vi "Dashboard Main.vi"() -> ()   [LabVIEW 2013]
uses:
  <vilib>/event_ctls.llb/eventvkey.ctl
  <vilib>/Rock Robotics/WPI/Dashboard/WPI_DashboardLogging Global.vi
  <vilib>/Utility/config.llb/Write Key (String).vi
  <vilib>/Utility/config.llb/Write Key (I32).vi
  <vilib>/Utility/config.llb/NI_LVConfig.lvlib
panel:
  out "fps":dbl format="%#.1g"
  out "Mbps":dbl format="%#.1g"
  out "Mbps 2":bool
  in  "DB Camera Config":bool
  out "Image Message":string="Timeout in Camera Communications"
  in  "Rec Mode":enum32{"Stop", "Record", "Playback"}(radio)
  in  "Dashboard Tab":T1(tab)
  in  "Encoder":dbl
  out "Compressor On/Off":bool
  in  "Camera Settings":T2={"Frame Rate"=30, "Compression"=30, "Size"=1} {"Frame Rate" scale=1.0..30.0; "Size" items=["640x480", "320x240", "160x120"]}
  out "MotorSliders R":cluster{"MotorSlide1":dbl, "MotorSlide2":dbl} {"MotorSlide2" scale=-1.0..1.0 scale format="%#_2e"; "MotorSlide1" scale=-1.0..1.0 scale format="%#_2e"}
  out "MotorChart R":cluster{"Numeric":dbl, "Numeric":dbl}(graph)
  out "MotorSliders L":T3 {"MotorSlide4 2" scale=0.0..14.0 scale format="%#_2e"; "MotorSlide2" scale=-1.0..1.0 scale format="%#_2e"; "MotorSlide1" scale=-1.0..1.0 scale format="%#_2e"}
  out "MotorChart L":T4(graph)
  out "JS1 Z":dbl(slide) scale=-1.0..1.0 scale format="%#_2e"
  out "Joystick 1":cluster{"X":dbl, "Y":dbl}[](graph)
  out "JS Buttons 1":T5
  out "JS2 Z":dbl(slide) scale=-1.0..1.0 scale format="%#_2e"
  out "Joystick 2":cluster{"X":dbl, "Y":dbl}[](graph)
  out "JS Buttons 2":T5
  out "Mode":T6(ring)=enum."Auto Disabled"
  out "Camera IP":string
  out "LED 1":bool
  in  "Throttle":dbl
  in  "Slider 1":dbl(slide) scale=0.0..100.0
  in  "Checkbox 2":bool
  in  "Checkbox 1":bool
  in  "Test Slider":dbl(slide) scale=0.0..100.0 scale format="%#_3g"
  in  "On/Off":bool caption="Solenoid"
  in  "Test Name":u16(ring) items=["Select the test to run...", "Example Test", "-------------------------------", "List of tests is built in robot code.", "Replace with your own automated tests."]
  in  "Test Tree":string(tree)
  in  "Motor":cluster{"Value":dbl, "Enable":bool} {"Value" scale=-1.0..1.0 scale format="%#_3g"}
  out "Progress":T7 {"Test Progress" scale=0.0..100.0}
  in  "Rev/Fwd":cluster{"Forward":bool, "Reverse":bool}
  in  "Test Ring":u16(ring) items=["Auto", "Fixed indoor", "Fixed outdoor 1", "Fixed outdoor 2", "Fixed fluorescent 1", "Fixed fluorescent 2", "Hold current"]
  in  "Listbox":i32(listbox)
  out "Tree":string(tree)
  out "Camera Image":T8(plugin-control)
  in  "Enable":bool
  # "Left"
  # "Front"
  # "Right"
  # "Battery"
  # "Customize by placing controls and indicators here and name to\nmatch Dashboard Variables on robot."
  # "This tab is a great place for autonomous settings and validation.\nCustomize by placing controls and indicators here and name to\nmatch Dashboard Variables on robot."
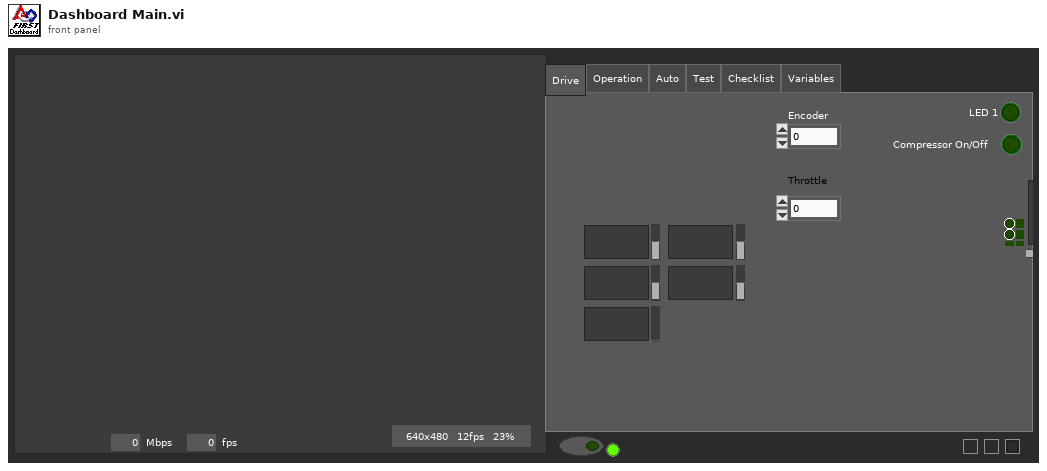
[diagram p1: front panel]
types:
  T1 = enum32{"Drive", "Operation", "Auto", "Test", "Checklist", "Variables"}
  T2 = cluster{"Frame Rate":i32, "Compression":i32, "Size":u16}
  T3 = cluster{"MotorSlide1":dbl, "MotorSlide2":dbl, "MotorSlide4 2":dbl}
  T4 = cluster{"Numeric":dbl, "Numeric":dbl, "Battery":sgl}
  T5 = cluster{bool, bool, bool, bool, bool, bool, bool, bool, bool, bool, bool, bool}
  T6 = enum8{"Tele-Op Disabled", "Tele-Op Enabled", "Auto Disabled", "Auto Enabled", "Test Disabled", "Test Enabled", ""}
  T7 = cluster{"Test Progress":u8, "Test Progress Text":string}
  T8 = typedef "IMAQ Image.ctl" = refnum<image>
  T9 = typedef "Image Type" = u32
  T10 = cluster{"Digital Inputs":bool[], "Digital Outputs":bool[]}
  T11 = cluster{"Competition mode":bool, "Robot Link":bool, "Autonomous":bool, "Enabled":bool, "E-Stop":bool, "Simulated":bool, "TestMode":bool, "Docked Window":bool}
  T12 = cluster{"Boolean Array[0]":bool, "Boolean Array[1]":bool, "Boolean Array[2]":bool, "Boolean Array[3]":bool, "Boolean Array[4]":bool, "Boolean Array[5]":bool, "Boolean Array[6]":bool, "Boolean Array[7]":bool, "Boolean Array[8]":bool, "Boolean Array[9]":bool, "Boolean Array[10]":bool, "Boolean Array[11]":bool}
  T13 = typedef "NI_LVConfig.lvlib/Config Data RefNum.ctl" = refnum<k1>
  T14 = typedef "eventvkey.ctl" = enum16{"ASCII", "Enter", "Return", "Shift", "Ctrl", "Alt", "Cmd", "Opt", "Caps", "NumLock", "Clear", "Break", "Up", "Down", "Left", "Right", "Insert", "Delete", "Home", "End", "PageUp", "PageDown", "Escape", "Help", "Pause", "ScrollLock", "F1", "F2", "F3", "F4", "F5", "F6", "F7", "F8", "F9", "F10", "F11", "F12", "F13", "F14", "F15", "F16", "F17", "F18", "F19", "F20", "F21", "F22", "F23", "F24", "Play", "VolumeUp", "VolumeDown", "Mute", "Two Byte Char"}
  T15 = cluster{"Image Size":bool, "Image Type":bool, "Pixel Value":bool, "ROI Information":bool, "Zoom Factor":bool}
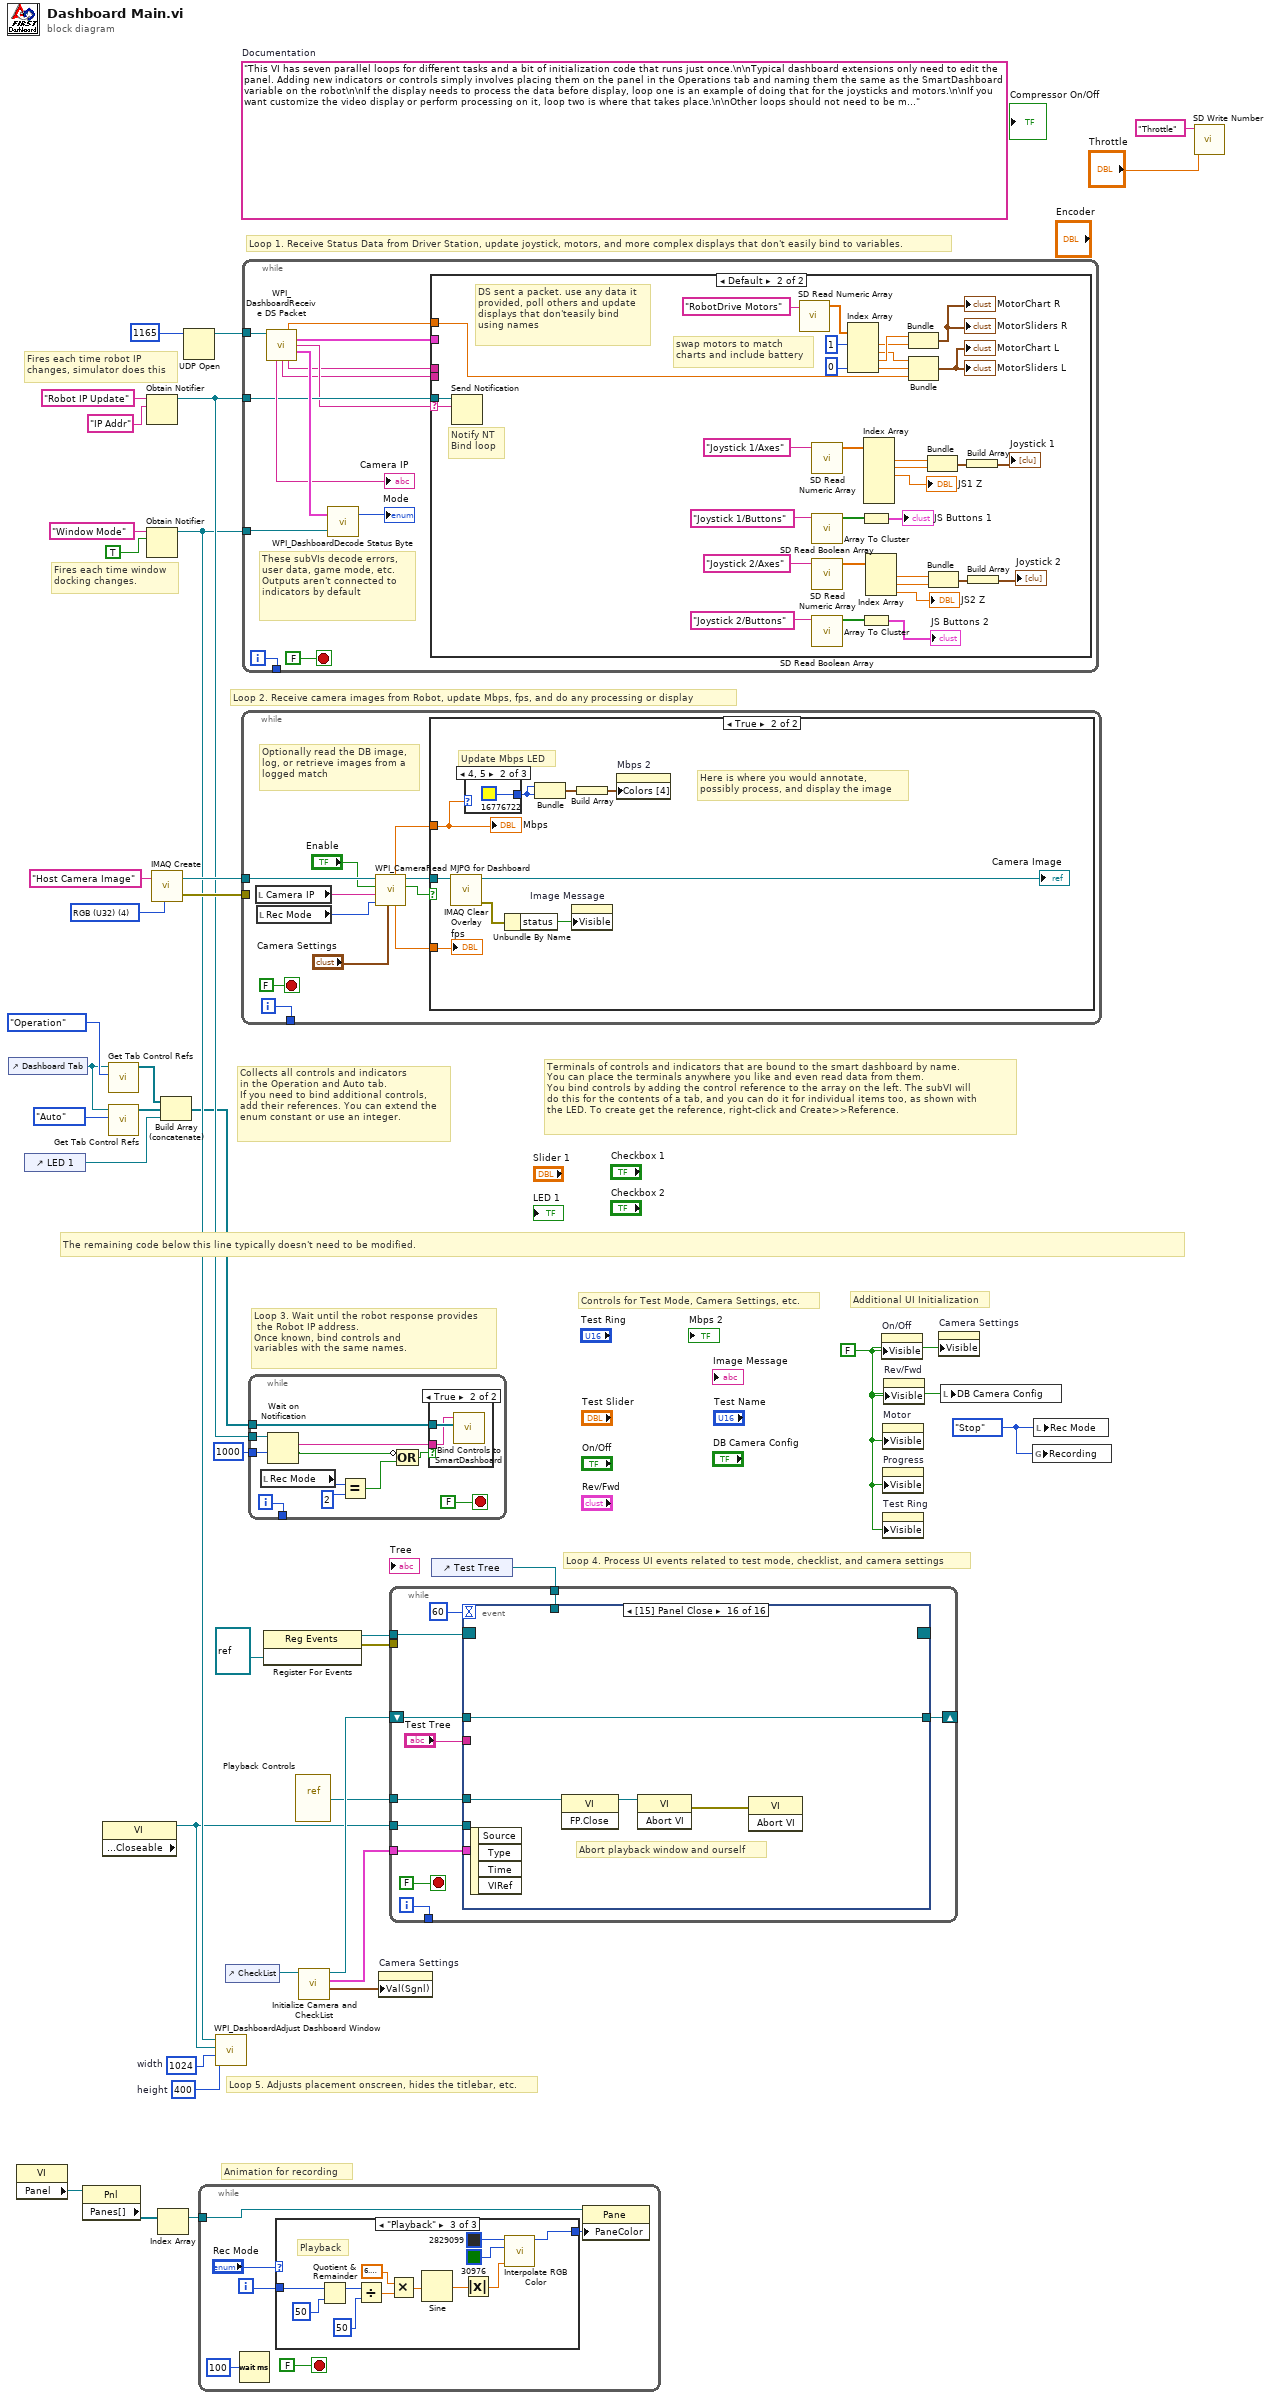
[diagram p0: block diagram]
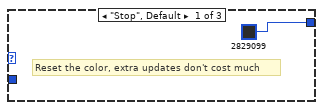
[diagram p2: hidden frame]
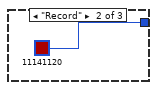
[diagram p3: hidden frame]
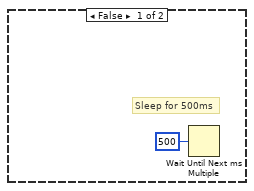
[diagram p5: hidden frame]
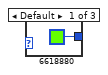
[diagram p6: hidden frame]
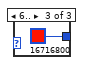
[diagram p7: hidden frame]
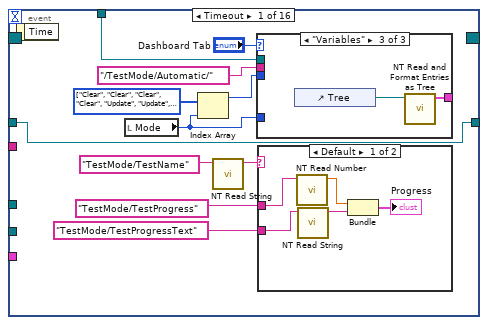
[diagram p8: hidden frame]
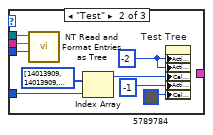
[diagram p10: hidden frame]
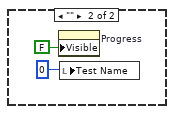
[diagram p11: hidden frame]
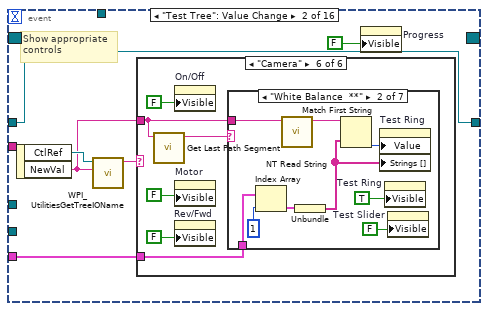
[diagram p12: hidden frame]
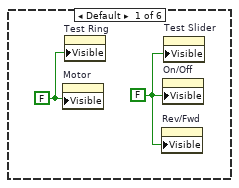
[diagram p13: hidden frame]
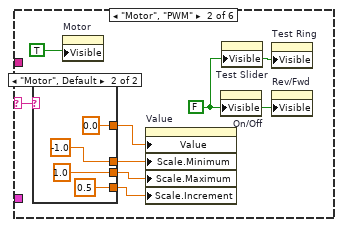
[diagram p14: hidden frame]
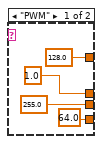
[diagram p15: hidden frame]
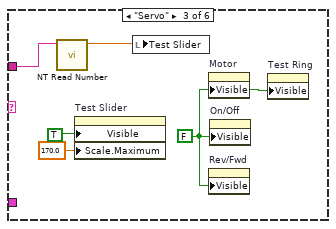
[diagram p16: hidden frame]
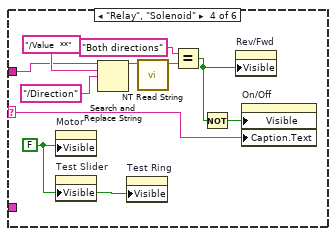
[diagram p17: hidden frame]
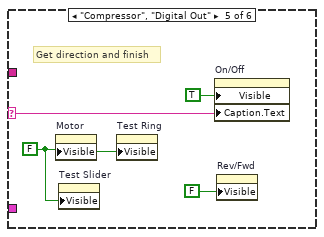
[diagram p18: hidden frame]
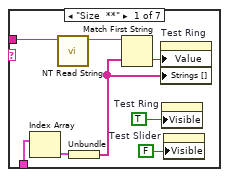
[diagram p19: hidden frame]
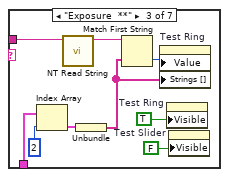
[diagram p20: hidden frame]
diagram:
  w10 = enum32{"Stop", "Record", "Playback"}."Stop" ("Rec Mode")
  w13 = 400  # height
  w14 = 1024  # width
  w27 = FALSE ("Visible")
  (unwired) "This VI has seven parallel loops for different tasks and a bit of initialization code that runs just once.\n\nTypical dashboard extensions only need to edit the panel. Adding new indicators or controls simply involves placing them on the panel in the Operations tab and naming them the same as the SmartDashboard variable on the robot\n\nIf the display needs to process the data before display, loop one is an example of doing that for the joysticks and motors.\n\nIf you want customize the video display or perform processing on it, loop two is where that takes place.\n\nOther loops should not need to be modified. They are pretty standard, and document the task they perform."  # Documentation
  w37 = T9 4 items=["Grayscale (U8)", "Grayscale (I16)", "Grayscale (SGL)", "Complex (CSG)", "RGB (U32)", "HSL (U32)", "RGB (U64)"] ("Image Type")
  # "Controls for Test Mode, Camera Settings, etc."
  # "Additional UI Initialization"
  # "Animation for recording"
  # "Fires each time robot IP\nchanges, simulator does this"
  # "Fires each time window\ndocking changes."
  # "Collects all controls and indicators\nin the Operation and Auto tab.\nIf you need to bind additional controls,\nadd their references. You can extend the\nenum constant or use an integer."
  # "The remaining code below this line typically doesn't need to be modified."
  # "Loop 4. Process UI events related to test mode, checklist, and camera settings"
  # "Terminals of controls and indicators that are bound to the smart dashboard by name.\nYou can place the terminals anywhere you like and even read data from them.\nYou bind controls by adding the control reference to the array on the left. The subVI will\ndo this for the contents of a tab, and you can do it for individual items too, as shown with\nthe LED. To create get the reference, right-click and Create>>Reference."
  # "Loop 3. Wait until the robot response provides\n the Robot IP address.\nOnce known, bind controls and\nvariables with the same names."
  # "Loop 5. Adjusts placement onscreen, hides the titlebar, etc."
  # "Loop 1. Receive Status Data from Driver Station, update joystick, motors, and more complex displays that don't easily bind to variables."
  # "Loop 2. Receive camera images from Robot, update Mbps, fps, and do any processing or display"
  n1 = control-ref of="Dashboard Tab"() -> (w8:refnum<vi>)
  n2 = property class="VI"() -> ("Panel"=w21:refnum<vi>)  [unwired: 2 in, 2 out]
  n3 = control-ref of="LED 1"() -> (w3:refnum<vi>)
  n4 = property class="Pnl"(reference=w21) -> ("Panes[]"=w22:refnum<vi>[])  [unwired: 1 in, 2 out]
  n5 = property class="VI" props=["Front Panel.Closeable"]() -> (reference out=w9:refnum<vi>)  [unwired: 2 in, 2 out]
  n6 = call <vilib>:"Get Tab Control Refs.vi"("Page Index"=T1."Operation" ("Dashboard Tab"), "TabControl in"=w8) -> ("ControlsOnPage"=w6:refnum<vi>[])  [unwired: 9 in]
  n7 = call <vilib>:"Get Tab Control Refs.vi"("Page Index"=T1."Auto" ("Dashboard Tab"), "TabControl in"=w8) -> ("ControlsOnPage"=w7:refnum<vi>[])  [unwired: 9 in]
  n8 = Obtain Notifier(name (unnamed)="Robot IP Update", notification data type="IP Addr" ("name (unnamed)")) -> (notifier out=w31:refnum<notifier>)  [unwired: 2 in, 2 out]
  n9 = Obtain Notifier(name (unnamed)="Window Mode", notification data type=TRUE) -> (notifier out=w12:refnum<notifier>)  [unwired: 2 in, 2 out]
  n10 = call "IMAQ Create"("Image Name"="Host Camera Image", "Image Type"=w37) -> ("New Image"=w35:T8, "error out"=w34:errorcluster)  [unwired: 2 in, 1 out]
  n11 = Index Array(array=w22) -> (element=w20:refnum<vi>)  [unwired: 1 in]
  n12 = Build Array (concatenate)(w6, w7, w3) -> (w5:refnum<vi>[])
  n13 = UDP Open(11:u16 1165 ("port")) -> (port=w38:refnum<k16>)  [unwired: 2 in, 4 out]
  n14 = while {
    tunnel: w20 -> [w41]
    i -> [w44]
    stop <- FALSE stop-if-true
    n15 = Wait (ms)(milliseconds to wait=u32 100) -> ()  [unwired: 1 out]
    n16 = case shown="\"Playback\"" "Rec Mode" {
      tunnel: w44 -> [_ _ w59]
      tunnel: [u32 2829099 ("Base Color") u32 11141120 ("Target Color") w48] -> w40
      frame "Stop", Default {
        # "Reset the color, extra updates don't cost much"
      }
      frame "Record" {
      }
      frame "Playback" {
        # "Playback"
        n17 = Quotient & Remainder(x=w59, y=u32 50 ("milliseconds to wait")) -> (x-y*floor(x/y)=w55:u32)  [unwired: 1 out]
        n18 = Divide(x=w55, y=u32 50 ("milliseconds to wait")) -> (x/y=w52:dbl)
        n19 = Multiply(x=6.283185307179586, y=w52) -> (x*y=w57:dbl)
        n20 = Sine(x=w57) -> (sin(x)=w56:dbl)
        n21 = Absolute Value(x=w56) -> (abs(x)=w49:dbl)
        n22 = call "Interpolate RGB Color.vi"("Proportion"=w49, "Target Color"=u32 30976, "Base Color"=u32 2829099) -> ("Result Color"=w48:u32)  [unwired: 8 in]
      }
    }
    n23 = property class="Pane"(reference=w41, "PaneColor"=w40) -> ()  [unwired: 1 in, 2 out]
  }
  n24 = call <vilib>:"WPI_DashboardAdjust Dashboard Window.vi"("height"=w13, "width"=w14, "reference in"=w9, "Notifier in"=w12) -> ()  [unwired: 8 in]
  n25 = control-ref of="CheckList"() -> (w11:refnum<vi>)
  n26 = while {
    tunnel: w35 -> [w68]
    tunnel: w34 -> [_]
    tunnel: [w69] -> _
    i -> [w69]
    stop <- FALSE stop-if-true
    # "Optionally read the DB image,\nlog, or retrieve images from a\nlogged match"
    n27 = local read "Camera IP"() -> (w61:string)
    n28 = local read "Rec Mode"() -> (w60:enum32{"Stop", "Record", "Playback"})
    n29 = call <vilib>:"WPI_CameraRead MJPG for Dashboard.vi"("Camera Settings"="Camera Settings", "Rec Mode"=w60, "Camera IP"=w61, "Enable"="Enable", "Refnum in"=w68) -> ("Active"=w65:bool, "Refnum out"=w67:T8, "FPS"=w64:dbl, "Bandwidth (Mbps)"=w63:dbl)  [unwired: 3 in]
    n30 = case shown="True" w65 {
      tunnel: w67 -> [_ w75]
      tunnel: w63 -> [_ w74]
      tunnel: w64 -> [_ w72]
      frame False {
        # "Sleep for 500ms"
        n31 = Wait Until Next ms Multiple(millisecond multiple=u32 500) -> ()  [unwired: 1 out]
      }
      frame True {
        # "Here is where you would annotate,\npossibly process, and display the image"
        # "Update Mbps LED"
        n32 = call "IMAQ Clear Overlay"("Image"=w75) -> ("error out"=w79:errorcluster, "Image Out"=→"Camera Image":T8)  [unwired: 2 in, 7 out]
        n33 = case shown="4, 5" w74 {
          tunnel: [u32 6618880 ("Color Box") u32 16776722 ("Color Box") u32 16716800 ("Color Box")] -> w76
          frame Default {
          }
          frame 4, 5 {
          }
          frame 6.. {
          }
        }
        n34 = Unbundle By Name(w79) -> ("status"=w80:bool)
        n35 = Bundle("Color Box"=w76, "Color Box"=w76) -> (w78:cluster{"Color Box":u32, "Color Box":u32})  [unwired: 1 out]
        n36 = property on="Image Message" class="Str"("Visible"=w80) -> ()  [unwired: 2 in, 2 out]
        n37 = Build Array(w78) -> (w77:cluster{"Color Box":u32, "Color Box":u32}[])
        n38 = property on="Mbps 2" class="Bool (strict)"("Colors [4]"=w77) -> ()  [unwired: 2 in, 2 out]
        "Mbps" <- w74
        "fps" <- w72
      }
    }
  }
  n39 = while {
    tunnel: w38 -> [w94]
    tunnel: w31 -> [w89]
    tunnel: w12 -> [w93]
    tunnel: [w90] -> _
    i -> [w90]
    stop <- FALSE stop-if-true
    # "These subVIs decode errors, user data, game mode, etc.\nOutputs aren't connected to indicators by default"
    n40 = call <vilib>:"WPI_DashboardReceive DS Packet.vi"("Recv Socket"=w94) -> ("Battery"=w84:sgl, "Driver Station"=w85:T10, "Robot IP Address"=w88:string, "Status"=w95:T11, "Camera IP Address"=→"Camera IP":string, "Low Priority User Data"=w87:string, "High Priority User Data"=w86:string)  [unwired: 1 in, 7 out]
    n41 = call <vilib>:"WPI_DashboardDecode Status Byte.vi"("Window Mode Notifier"=w93, "Status"=w95) -> ("Mode"=→"Mode":T6)  [unwired: 1 out]
    n42 = case shown="Default" w88 {
      selector: w88 -> [_ w107]
      tunnel: w89 -> [_ w108]
      tunnel: w87 -> [_ _]
      tunnel: w86 -> [_ _]
      tunnel: w85 -> [_ _]
      tunnel: w84 -> [_ w106]
      frame "0.0.0.0" {
        # "DS not sending packets, or no robot exists yet.\nDon't poll the variables"
      }
      frame Default {
        # "Notify NT\nBind loop"
        # "DS sent a packet. use any data it\nprovided, poll others and update\ndisplays that don'teasily bind\nusing names"
        # "swap motors to match\ncharts and include battery"
        n43 = Send Notification(notification=w107, notifier=w108) -> ()  [unwired: 1 in, 2 out]
        n44 = call <vilib>:"SD Read Numeric Array.vi"("Name"="RobotDrive Motors") -> ("Numeric Array"=w105:dbl[])  [unwired: 8 in, 2 out]
        n45 = call <vilib>:"SD Read Numeric Array.vi"("Name"="Joystick 1/Axes") -> ("Numeric Array"=w124:dbl[])  [unwired: 8 in, 2 out]
        n46 = call <vilib>:"SD Read Boolean Array.vi"("Name"="Joystick 1/Buttons") -> ("Boolean Array"=w126:bool[])  [unwired: 8 in, 2 out]
        n47 = call <vilib>:"SD Read Numeric Array.vi"("Name"="Joystick 2/Axes") -> ("Numeric Array"=w118:dbl[])  [unwired: 8 in, 2 out]
        n48 = call <vilib>:"SD Read Boolean Array.vi"("Name"="Joystick 2/Buttons") -> ("Boolean Array"=w117:bool[])  [unwired: 8 in, 2 out]
        n49 = Index Array(array=w105, index #1=1, index #4=0) -> (element #1=w101:dbl, element #2=w100:dbl, element #3=w102:dbl, element #4=w97:dbl)  [unwired: 2 in]
        n50 = Array To Cluster(array=w126) -> (cluster=→"JS Buttons 1":T12)
        n51 = Array To Cluster(array=w117) -> (cluster=→"JS Buttons 2":T12)
        n52 = Index Array(array=w124) -> (element #1=w121:dbl, element #2=w122:dbl, element #3=→"JS1 Z":dbl)  [unwired: 6 in, 3 out]
        n53 = Index Array(array=w118) -> (element #1=w113:dbl, element #2=w112:dbl, element #3=→"JS2 Z":dbl)  [unwired: 3 in]
        n54 = Bundle("Numeric"=w102, "Numeric"=w101) -> (→"MotorChart R" →"MotorSliders R":cluster{"Numeric":dbl, "Numeric":dbl})  [unwired: 1 in]
        n55 = Bundle("Numeric"=w100, "Numeric"=w97, "Battery"=w106) -> (→"MotorChart L" →"MotorSliders L":T4)  [unwired: 1 in]
        n56 = Bundle("Numeric"=w121, "Numeric"=w122) -> (w120:cluster{"Numeric":dbl, "Numeric":dbl})  [unwired: 1 in]
        n57 = Bundle("Numeric"=w113, "Numeric"=w112) -> (w114:cluster{"Numeric":dbl, "Numeric":dbl})  [unwired: 1 in]
        n58 = Build Array(w120) -> (→"Joystick 1":cluster{"Numeric":dbl, "Numeric":dbl}[])
        n59 = Build Array(w114) -> (→"Joystick 2":cluster{"Numeric":dbl, "Numeric":dbl}[])
      }
    }
  }
  n60 = while {
    tunnel: w5 -> [w140]
    tunnel: w31 -> [w138]
    tunnel: [w136] -> _
    tunnel: u32 1000 ("milliseconds to wait") -> [w135]
    i -> [w136]
    stop <- FALSE stop-if-true
    n61 = local read "Rec Mode"() -> (w131:enum32{"Stop", "Record", "Playback"})
    n62 = Wait on Notification(notifier=w138, timeout in ms (-1)=w135) -> (notification=w137:string, timed out?=w133:bool)  [unwired: 2 in, 2 out]
    n63 = Equal?(x=w131, y=u16 2 ("Rec Mode")) -> (x = y?=w132:bool)
    n64 = Compound Arithmetic op=OR(invert w133, w132) -> (w134:bool)
    n65 = case shown="True" w134 {
      tunnel: w140 -> [_ w142]
      tunnel: w137 -> [_ w141]
      frame False {
      }
      frame True {
        n66 = call <vilib>:"Bind Controls to SmartDashboard.vi"("Bound Control Refs"=w142, "Server IP Address"=w141) -> ()  [unwired: 10 in]
      }
    }
  }
  n67 = register-events(refnum<vi> refnum) -> (reference out=w18:refnum<event-registration>, error out=w17:errorcluster)  [unwired: 2 in]
  n68 = vi-ref "Playback Controls.vi"() -> (w19:refnum<vi>)
  n69 = call "Initialize Camera and CheckList.vi"("ListBox in"=w11) -> ("Cluster"=w25:cluster{"value":i32, "value":i32, "index":i32}, "Array"=w26:cluster{string[]}[], "File Refnum"=w24:T13)  [unwired: 8 in]
  n70 = property on="Camera Settings" class="Clust (strict)"("Val(Sgnl)"=w25) -> ()  [unwired: 2 in, 2 out]
  n71 = control-ref of="Test Tree"() -> (w23:refnum<vi>)
  n72 = while {
    tunnel: w26 -> [w150]
    shift-right: [w149] -> _
    shift-left: w24 -> [w148]
    tunnel: [w147] -> _
    tunnel: w23 -> [w146]
    tunnel: w19 -> [w145]
    tunnel: w18 -> [w144]
    tunnel: w17 -> [_]
    tunnel: w9 -> [w143]
    i -> [w147]
    stop <- FALSE stop-if-true
    n73 = event shown="[15] Panel Close" {
      selector: w144 -> [_ _ _ _ _ _ _ _ _ _ _ _ _ _ _ _]
      dyn-events: [_ _ _ _ _ _ _ _ _ _ _ _ _ w388 _ _] -> _
      timeout: u32 60 ("milliseconds to wait") -> [_ _ _ _ _ _ _ _ _ _ _ _ _ _ _ _]
      tunnel: w146 -> [w160 _ _ _ _ _ _ _ _ _ _ _ _ _ _ _]
      tunnel: "Test Tree" -> [_ _ _ _ _ _ _ _ w357 w365 w367 w371 w379 _ _ _]
      tunnel: w150 -> [_ w184 _ _ _ _ w321 w351 _ _ _ _ _ _ _ _]
      tunnel: [w154 w183 w282 w287 w295 w307 w320 w344 w356 w363 w366 w370 w378 w390 w404 w405] -> w149
      tunnel: w148 -> [w154 w183 w282 w287 w295 w307 w319 w344 w356 w363 w366 w370 w378 w390 w404 w405]
      tunnel: w145 -> [_ _ _ _ _ _ _ _ _ _ _ _ _ w391 _ w408]
      tunnel: w143 -> [_ _ _ _ _ _ _ _ _ _ _ _ _ w386 _ _]
      event Timeout {
        w159 = enum16{"Update", "Clear"}[] [enum."Clear", enum."Clear", enum."Clear", enum."Clear", enum."Update", enum."Update", enum."Clear"] items=["Update", "Clear"]
        n74 = event-data() -> ()  [unwired: 1 in, 1 out]
        n75 = local read "Mode"() -> (w157:T6)
        n76 = Index Array(array=w159, index=w157) -> (element=w158:enum16{"Update", "Clear"})
        n77 = call <vilib>:"NT Read String.vi"("Name"="TestMode/TestName") -> ("String"=w163:string)  [unwired: 9 in, 1 out]
        n78 = case shown="\"Variables\"" "Dashboard Tab" {
          tunnel: w160 -> [_ w173 _]
          tunnel: "/TestMode/Automatic/" ("Name Pattern") -> [_ w172 _]
          tunnel: w158 -> [_ w171 _]
          tunnel: w157 -> [_ w169 _]
          tunnel: [_ _ w175] -> _
          frame "Operation", Default {
          }
          frame "Test" {
            w168 = -2 ("Active Item:Row Number")
            n79 = call <vilib>:"NT Read and Format Entries as Tree.vi"("Operation"=w171, "Name Pattern"=w172, "Tree Refnum"=w173) -> ()  [unwired: 7 in, 2 out]
            n80 = Index Array(array=u32[] [14013909, 14013909, 14013909, 14013909, 14013909, 16777215, 14013909], index=w169) -> (element=w167:u32)
            n81 = property on="Test Tree" class="Tree (strict)"("Active Item Row Number"=w168, "ActiveColNum"=w168, "CellBG"=w167, "Active Item Row Number"=-1 ("Active Item:Row Number"), "CellBG"=u32 5789784 ("Color Box")) -> ()  [unwired: 2 in, 2 out]
          }
          frame "Variables" {
            n82 = control-ref of="Tree"() -> (w174:refnum<vi>)
            n83 = call <vilib>:"NT Read and Format Entries as Tree.vi"("Tree Refnum"=w174) -> ("Formatted Strings"=w175:cluster{"Name":string, "Value":string}[])  [unwired: 9 in, 1 out]
          }
        }
        n84 = case shown="Default" w163 {
          tunnel: "TestMode/TestProgress" ("Name") -> [w177 _]
          tunnel: "TestMode/TestProgressText" ("Name") -> [w176 _]
          frame Default {
            n85 = call <vilib>:"NT Read Number.vi"("Name"=w177) -> ("Numeric"=w178:dbl)  [unwired: 9 in, 1 out]
            n86 = call <vilib>:"NT Read String.vi"("Name"=w176) -> ("String"=w179:string)  [unwired: 9 in, 1 out]
            n87 = Bundle("Numeric"=w178, "String"=w179) -> (→"Progress":cluster{"Numeric":dbl, "String":string})  [unwired: 1 in]
          }
          frame "" {
            n88 = property on="Progress" class="Clust (strict)"("Visible"=FALSE) -> ()  [unwired: 2 in, 2 out]
            n89 = local write "Test Name"(u16 0) -> ()
          }
        }
      }
      event "Test Tree": Value Change {
        # "Show appropriate\ncontrols"
        n90 = event-data() -> ("CtlRef"=w187:refnum<vi>, "NewVal"=w185:string)  [unwired: 1 in]
        n91 = call <vilib>:"WPI_UtilitiesGetTreeIOName.vi"("NewVal"=w185, "TreeControl in"=w187) -> ("I/O Name"=w188:string)  [unwired: 9 in]
        n92 = case shown="\"Camera\"" w188 {
          selector: w188 -> [_ w195 _ w213 w222 _]
          tunnel: w185 -> [_ _ w210 w212 _ w229]
          tunnel: w184 -> [_ _ _ _ _ w228]
          frame Default {
            w190 = FALSE ("Visible")
            w189 = FALSE ("Visible")
            n93 = property on="Motor" class="Clust (strict)"("Visible"=w189) -> ()  [unwired: 2 in, 2 out]
            n94 = property on="Test Ring" class="Ring (strict)"("Visible"=w189) -> ()  [unwired: 2 in, 2 out]
            n95 = property on="Rev/Fwd" class="Clust (strict)"("Visible"=w190) -> ()  [unwired: 2 in, 2 out]
            n96 = property on="On/Off" class="Bool (strict)"("Visible"=w190) -> ()  [unwired: 2 in, 2 out]
            n97 = property on="Test Slider" class="Slide (strict)"("Visible"=w190) -> ()  [unwired: 2 in, 2 out]
          }
          frame "Motor", "PWM" {
            w196 = FALSE ("Visible")
            n98 = case shown="\"Motor\", Default" w195 {
              tunnel: [1.0 ("Value") -1.0 ("Value")] -> w194
              tunnel: [255.0 ("Value") 1.0 ("Value")] -> w193
              tunnel: [128.0 ("Value") 0.0 ("Value")] -> w192
              tunnel: [64.0 ("Value") 0.5 ("Value")] -> w191
              frame "PWM" {
              }
              frame "Motor", Default {
              }
            }
            n99 = property on="Motor" class="Clust (strict)"("Visible"=TRUE) -> ()  [unwired: 2 in, 2 out]
            n100 = property on="Value" class="Slide (strict)"("Value"=w192, "Scale.Minimum"=w194, "Scale.Maximum"=w193, "Scale.Increment"=w191) -> ()  [unwired: 2 in, 2 out]
            n101 = property on="On/Off" class="Bool (strict)"("Visible"=w196) -> ()  [unwired: 2 in, 2 out]
            n102 = property on="Test Slider" class="Slide (strict)"("Visible"=w196) -> ()  [unwired: 2 in, 2 out]
            n103 = property on="Test Ring" class="Ring (strict)"("Visible"=w196) -> ()  [unwired: 2 in, 2 out]
            n104 = property on="Rev/Fwd" class="Clust (strict)"("Visible"=w196) -> ()  [unwired: 2 in, 2 out]
          }
          frame "Servo" {
            w208 = FALSE ("Visible")
            n105 = call <vilib>:"NT Read Number.vi"("Name"=w210) -> ("Numeric"=w209:dbl)  [unwired: 9 in, 1 out]
            n106 = property on="Test Slider" class="Slide (strict)"("Visible"=TRUE, "Scale.Maximum"=170.0 ("Scale.Range:Maximum")) -> ()  [unwired: 2 in, 2 out]
            n107 = local write "Test Slider"(w209) -> ()
            n108 = property on="Motor" class="Clust (strict)"("Visible"=w208) -> ()  [unwired: 2 in, 2 out]
            n109 = property on="Rev/Fwd" class="Clust (strict)"("Visible"=w208) -> ()  [unwired: 2 in, 2 out]
            n110 = property on="On/Off" class="Bool (strict)"("Visible"=w208) -> ()  [unwired: 2 in, 2 out]
            n111 = property on="Test Ring" class="Ring (strict)"("Visible"=w208) -> ()  [unwired: 2 in, 2 out]
          }
          frame "Relay", "Solenoid" {
            w211 = FALSE ("Visible")
            n112 = property on="Motor" class="Clust (strict)"("Visible"=w211) -> ()  [unwired: 2 in, 2 out]
            n113 = property on="Test Slider" class="Slide (strict)"("Visible"=w211) -> ()  [unwired: 2 in, 2 out]
            n114 = Search and Replace String(input string=w212, search string="/Value  **", replace string="/Direction") -> (result string=w218:string)  [unwired: 5 in, 3 out]
            n115 = property on="Test Ring" class="Ring (strict)"("Visible"=w211) -> ()  [unwired: 2 in, 2 out]
            n116 = call <vilib>:"NT Read String.vi"("Name"=w218) -> ("String"=w216:string)  [unwired: 9 in, 1 out]
            n117 = Equal?(x="Both directions", y=w216) -> (x = y?=w214:bool)
            n118 = Not(x=w214) -> (.not. x?=w215:bool)
            n119 = property on="Rev/Fwd" class="Clust (strict)"("Visible"=w214) -> ()  [unwired: 2 in, 2 out]
            n120 = property on="On/Off" class="Bool (strict)"("Visible"=w215, "Caption.Text"=w213) -> ()  [unwired: 2 in, 2 out]
          }
          frame "Compressor", "Digital Out" {
            w221 = FALSE ("Visible")
            # "Get direction and finish"
            n121 = property on="Motor" class="Clust (strict)"("Visible"=w221) -> ()  [unwired: 2 in, 2 out]
            n122 = property on="Test Slider" class="Slide (strict)"("Visible"=w221) -> ()  [unwired: 2 in, 2 out]
            n123 = property on="Test Ring" class="Ring (strict)"("Visible"=w221) -> ()  [unwired: 2 in, 2 out]
            n124 = property on="On/Off" class="Bool (strict)"("Visible"=TRUE, "Caption.Text"=w222) -> ()  [unwired: 2 in, 2 out]
            n125 = property on="Rev/Fwd" class="Clust (strict)"("Visible"=FALSE) -> ()  [unwired: 2 in, 2 out]
          }
          frame "Camera" {
            n126 = call <vilib>:"Get Last Path Segment.vi"("String in"=w229) -> ("String out"=w230:string)  [unwired: 10 in]
            n127 = property on="On/Off" class="Bool (strict)"("Visible"=FALSE) -> ()  [unwired: 2 in, 2 out]
            n128 = property on="Motor" class="Clust (strict)"("Visible"=FALSE) -> ()  [unwired: 2 in, 2 out]
            n129 = property on="Rev/Fwd" class="Clust (strict)"("Visible"=FALSE) -> ()  [unwired: 2 in, 2 out]
            n130 = case shown="\"White Balance  **\"" w230 {
              tunnel: w229 -> [w236 w245 w254 w263 w272 _ w278]
              tunnel: w228 -> [w234 w242 w251 w260 w269 _ _]
              frame "Size  **" {
                n131 = Index Array(array=w234) -> (element=w233:cluster{string[]})  [unwired: 1 in]
                n132 = call <vilib>:"NT Read String.vi"("Name"=w236) -> ("String"=w235:string)  [unwired: 9 in, 1 out]
                n133 = Unbundle(w233) -> (w231:string[])
                n134 = Match First String(2:w231, 3:w235) -> (0:w232:i32)  [unwired: 1 out]
                n135 = property on="Test Ring" class="Ring (strict)"("Value"=w232, "Strings []"=w231) -> ()  [unwired: 2 in, 2 out]
                n136 = property on="Test Ring" class="Ring (strict)"("Visible"=TRUE) -> ()  [unwired: 2 in, 2 out]
                n137 = property on="Test Slider" class="Slide (strict)"("Visible"=FALSE) -> ()  [unwired: 2 in, 2 out]
              }
              frame "White Balance  **" {
                n138 = Index Array(array=w242, index=1) -> (element=w243:cluster{string[]})
                n139 = call <vilib>:"NT Read String.vi"("Name"=w245) -> ("String"=w244:string)  [unwired: 9 in, 1 out]
                n140 = Unbundle(w243) -> (w240:string[])
                n141 = Match First String(2:w240, 3:w244) -> (0:w239:i32)  [unwired: 1 out]
                n142 = property on="Test Ring" class="Ring (strict)"("Value"=w239, "Strings []"=w240) -> ()  [unwired: 2 in, 2 out]
                n143 = property on="Test Ring" class="Ring (strict)"("Visible"=TRUE) -> ()  [unwired: 2 in, 2 out]
                n144 = property on="Test Slider" class="Slide (strict)"("Visible"=FALSE) -> ()  [unwired: 2 in, 2 out]
              }
              frame "Exposure  **" {
                n145 = Index Array(array=w251, index=2) -> (element=w252:cluster{string[]})
                n146 = call <vilib>:"NT Read String.vi"("Name"=w254) -> ("String"=w253:string)  [unwired: 9 in, 1 out]
                n147 = Unbundle(w252) -> (w248:string[])
                n148 = Match First String(2:w248, 3:w253) -> (0:w249:i32)  [unwired: 1 out]
                n149 = property on="Test Ring" class="Ring (strict)"("Value"=w249, "Strings []"=w248) -> ()  [unwired: 2 in, 2 out]
                n150 = property on="Test Ring" class="Ring (strict)"("Visible"=TRUE) -> ()  [unwired: 2 in, 2 out]
                n151 = property on="Test Slider" class="Slide (strict)"("Visible"=FALSE) -> ()  [unwired: 2 in, 2 out]
              }
              frame "Exposure Priority  **" {
                n152 = Index Array(array=w260, index=3) -> (element=w261:cluster{string[]})
                n153 = call <vilib>:"NT Read String.vi"("Name"=w263) -> ("String"=w262:string)  [unwired: 9 in, 1 out]
                n154 = Unbundle(w261) -> (w257:string[])
                n155 = Match First String(2:w257, 3:w262) -> (0:w258:i32)  [unwired: 1 out]
                n156 = property on="Test Ring" class="Ring (strict)"("Value"=w258, "Strings []"=w257) -> ()  [unwired: 2 in, 2 out]
                n157 = property on="Test Ring" class="Ring (strict)"("Visible"=TRUE) -> ()  [unwired: 2 in, 2 out]
                n158 = property on="Test Slider" class="Slide (strict)"("Visible"=FALSE) -> ()  [unwired: 2 in, 2 out]
              }
              frame "Color Enable  **" {
                n159 = Index Array(array=w269, index=4) -> (element=w270:cluster{string[]})
                n160 = call <vilib>:"NT Read String.vi"("Name"=w272) -> ("String"=w271:string)  [unwired: 9 in, 1 out]
                n161 = Unbundle(w270) -> (w266:string[])
                n162 = Match First String(2:w266, 3:w271) -> (0:w267:i32)  [unwired: 1 out]
                n163 = property on="Test Ring" class="Ring (strict)"("Value"=w267, "Strings []"=w266) -> ()  [unwired: 2 in, 2 out]
                n164 = property on="Test Ring" class="Ring (strict)"("Visible"=TRUE) -> ()  [unwired: 2 in, 2 out]
                n165 = property on="Test Slider" class="Slide (strict)"("Visible"=FALSE) -> ()  [unwired: 2 in, 2 out]
              }
              frame Default {
                n166 = property on="Test Ring" class="Ring (strict)"("Visible"=FALSE) -> ()  [unwired: 2 in, 2 out]
                n167 = property on="Test Slider" class="Slide (strict)"("Visible"=FALSE) -> ()  [unwired: 2 in, 2 out]
              }
              frame "Brightness  **", "Color Level  **", "Compression  **", "FPS  **", "Sharpness  **" {
                n168 = call <vilib>:"NT Read Number.vi"("Name"=w278) -> ("Numeric"=w277:dbl)  [unwired: 9 in, 1 out]
                n169 = local write "Test Slider"(w277) -> ()
                n170 = property on="Test Slider" class="Slide (strict)"("Visible"=TRUE, "Scale.Maximum"=100.0 ("Scale.Range:Maximum")) -> ()  [unwired: 2 in, 2 out]
                n171 = property on="Test Ring" class="Ring (strict)"("Visible"=FALSE) -> ()  [unwired: 2 in, 2 out]
              }
            }
          }
        }
        n172 = property on="Progress" class="Clust (strict)"("Visible"=FALSE) -> ()  [unwired: 2 in, 2 out]
      }
      event "Test Name": Mouse Enter {
        # "Populate the ring with the list of tests"
        n173 = event-data() -> ()  [unwired: 1 in, 1 out]
        n174 = call <vilib>:"NT Read String Array.vi"("Name"="TestMode/TestList") -> ("String Array"=w286:string[])  [unwired: 9 in, 1 out]
        n175 = Build Array (concatenate)("Select the test to run...", w286) -> (w285:string[])
        n176 = property on="Test Name" class="Ring (strict)"("Strings []"=w285) -> ()  [unwired: 2 in, 2 out]
      }
      event "Test Name": Value Change {
        w288 = FALSE ("Visible")
        # "Tell the robot the test name to run"
        n177 = event-data() -> ("NewVal"=w292:u16)  [unwired: 1 in]
        n178 = property on="Test Name" class="Ring (strict)"() -> ("Strings []"=w293:string[])  [unwired: 2 in, 2 out]
        n179 = local write "Progress"(T7 {"Test Progress"=0, "Test Progress Text"=""} ("Progress")) -> ()
        n180 = Index Array(array=w293, index=w292) -> (element=w291:string)
        n181 = call <vilib>:"NT Write String.vi"("String"=w291, "Name"="TestMode/TestName") -> ()  [unwired: 9 in, 1 out]
        n182 = property on="Progress" class="Clust (strict)"("Visible"=TRUE) -> ()  [unwired: 2 in, 2 out]
        n183 = property on="Motor" class="Clust (strict)"("Visible"=w288) -> ()  [unwired: 2 in, 2 out]
        n184 = property on="Test Slider" class="Slide (strict)"("Visible"=w288) -> ()  [unwired: 2 in, 2 out]
        n185 = property on="On/Off" class="Bool (strict)"("Visible"=w288) -> ()  [unwired: 2 in, 2 out]
        n186 = property on="Rev/Fwd" class="Clust (strict)"("Visible"=w288) -> ()  [unwired: 2 in, 2 out]
        n187 = property on="Test Ring" class="Ring (strict)"("Visible"=w288) -> ()  [unwired: 2 in, 2 out]
      }
      event "Listbox": Double Click {
        n188 = event-data() -> ("PlatMods.Shift"=w296:bool, "Row"=w298:i32)  [unwired: 1 in]
        n189 = case shown="True" w296 {
          tunnel: w298 -> [w302 _]
          tunnel: 1 -> [w301 _]
          frame False {
            n190 = property on="Listbox" class="LstBox (strict)"() -> ("Item Symbols"=w300:i32[])  [unwired: 2 in, 2 out]
            n191 = Replace Array Subset(array=w300, new element=w301, index=w302) -> (w299:i32[])
            n192 = property on="Listbox" class="LstBox (strict)"("Item Symbols"=w299) -> ()  [unwired: 2 in, 2 out]
          }
          frame True {
            w303 = 0 ("Top Row")
            n193 = property on="Listbox" class="LstBox (strict)"() -> ("Number of Rows"=w305:u32)  [unwired: 2 in, 2 out]
            n194 = Initialize Array(0, w305) -> (w304:i32[])
            n195 = property on="Listbox" class="LstBox (strict)"("Top Row"=w303, "Value"=w303, "Item Symbols"=w304) -> ()  [unwired: 2 in, 2 out]
          }
        }
      }
      event "Listbox": Key Down {
        n196 = event-data() -> ("VKey"=w309:T14)  [unwired: 1 in]
        n197 = case shown="\"Left\", \"Right\"" w309 {
          selector: w309 -> [w314 _]
          tunnel: eventvkey."Left" ("VKey") -> [w312 _]
          frame "Left", "Right" {
            n198 = Equal?(x=w312, y=w314) -> (x = y?=w313:bool)
            n199 = Select(t=0, s=w313, f=1) -> (s? t:f=w315:i32)
            n200 = property on="Listbox" class="LstBox (strict)"() -> ("Item Symbols"=w318:i32[])  [unwired: 2 in, 2 out]
            n201 = Replace Array Subset(array=w318, new element=w315, index="Listbox") -> (w317:i32[])
            n202 = property on="Listbox" class="LstBox (strict)"("Item Symbols"=w317) -> ()  [unwired: 2 in, 2 out]
          }
          frame Default {
          }
        }
      }
      event "DB Camera Config": Value Change {
        n203 = event-data() -> ("NewVal"=w322:bool)  [unwired: 1 in]
        n204 = case shown="False" w322 {
          tunnel: w321 -> [w331 _]
          tunnel: [w324 w342] -> w320
          tunnel: w319 -> [w323 w342]
          frame False {
            w338 = "Camera"
            w341 = FALSE ("Visible")
            n205 = local read "Camera Settings"() -> (w330:T2)
            n206 = Index Array(array=w331) -> (element=w334:cluster{string[]})  [unwired: 1 in]
            n207 = Unbundle(w330) -> ("Frame Rate"=w329:i32, "Compression"=w328:i32, "Size"=w332:u16)
            n208 = Unbundle(w334) -> (w333:string[])
            n209 = Index Array(array=w333, index=w332) -> (element=w327:string)
            n210 = call-poly <vilib>:"Write Key.vi"("section"=w338, "value"=w327, "key"="Size", "refnum"=w323) -> ("refnum out"=w340:T13)  [unwired: 2 in, 5 out]
            n211 = call-poly <vilib>:"Write Key.vi"("section"=w338, "value"=w329, "key"="FrameRate", "refnum"=w340) -> ("refnum out"=w339:T13)  [unwired: 1 in, 6 out]
            n212 = property on="Camera Settings" class="Clust (strict)"("Visible"=w341) -> ()  [unwired: 2 in, 2 out]
            n213 = local write "DB Camera Config"(w341) -> ()
            n214 = call-poly <vilib>:"Write Key.vi"("section"=w338, "value"=w328, "key"="Compression", "refnum"=w339) -> ("refnum out"=w325:T13)  [unwired: 1 in, 6 out]
            n215 = call <vilib>:"Close Config Data.vi"("refnum"=w325) -> ("file path"=w326:path)  [unwired: 2 in, 8 out]
            n216 = call <vilib>:"Open Config Data.vi"("configuration file path"=w326) -> ("refnum"=w324:T13)  [unwired: 8 in, 2 out]
          }
          frame True {
            n217 = property on="Camera Settings" class="Clust (strict)"("Visible"=TRUE) -> ()  [unwired: 2 in, 2 out]
          }
        }
      }
      event "Camera Settings": Value Change {
        n218 = event-data() -> ("NewVal"=w355:T2)  [unwired: 1 in]
        n219 = Index Array(array=w351) -> (element=w350:cluster{string[]})  [unwired: 1 in]
        n220 = Unbundle(w355) -> ("Frame Rate"=w346:i32, "Compression"=w345:i32, "Size"=w348:u16)
        n221 = Unbundle(w350) -> (w349:string[])
        n222 = Index Array(array=w349, index=w348) -> (element=w347:string)
        n223 = Format Into String(format string="%s   %dfps   %d%%", w347, w346, w345) -> (resulting string=w352:string)  [unwired: 2 in, 1 out]
        n224 = Build Array(w352) -> (w353:string[])
        n225 = property on="DB Camera Config" class="Bool (strict)"("Strings [4]"=w353) -> ()  [unwired: 2 in, 2 out]
      }
      event "Motor.Enable": Value Change {
        n226 = event-data() -> ("NewVal"=w361:bool)  [unwired: 1 in]
        n227 = Unbundle("Motor") -> ("Value"=w360:dbl)  [unwired: 1 out]
        n228 = Select(t=w360, s=w361, f=0.0) -> (s? t:f=w358:dbl)
        n229 = call <vilib>:"NT Write Number.vi"("Numeric"=w358, "Name"=w357) -> ()  [unwired: 9 in, 1 out]
      }
      event "Test Slider": Value Change {
        n230 = event-data() -> ("NewVal"=w364:dbl)  [unwired: 1 in]
        n231 = call <vilib>:"NT Write Number.vi"("Numeric"=w364, "Name"=w365) -> ()  [unwired: 9 in, 1 out]
      }
      event "On/Off": Value Change {
        n232 = event-data() -> ("NewVal"=w369:bool)  [unwired: 1 in]
        n233 = Boolean To (0,1)(Boolean=w369) -> (0, 1=w368:i16)
        n234 = call <vilib>:"NT Write Number.vi"("Numeric"=w368, "Name"=w367) -> ()  [unwired: 9 in, 1 out]
      }
      event "Rev/Fwd": Value Change {
        n235 = event-data() -> ("NewVal.Forward"=w377:bool, "NewVal.Reverse"=w376:bool)  [unwired: 1 in]
        n236 = Boolean To (0,1)(Boolean=w377) -> (0, 1=w373:i16)
        n237 = Boolean To (0,1)(Boolean=w376) -> (0, 1=w375:i16)
        n238 = Negate(x=w375) -> (-x=w374:i16)
        n239 = Add(x=w373, y=w374) -> (x+y=w372:i16)
        n240 = call <vilib>:"NT Write Number.vi"("Numeric"=w372, "Name"=w371) -> ()  [unwired: 9 in, 1 out]
      }
      event "Test Ring": Value Change {
        n241 = event-data() -> ("NewVal"=w381:u16)  [unwired: 1 in]
        n242 = property on="Test Ring" class="Ring (strict)"() -> ("Strings []"=w382:string[])  [unwired: 2 in, 2 out]
        n243 = Index Array(array=w382, index=w381) -> (element=w380:string)
        n244 = call <vilib>:"NT Write String.vi"("String"=w380, "Name"=w379) -> ()  [unwired: 9 in, 1 out]
      }
      event "Rec Mode": Value Change {
        # "Update globals for recording mode and path to read log from.\nClear when logging and let NetworkTables set path for vision to\nuse."
        n245 = event-data() -> ("NewVal"=w392:enum32{"Stop", "Record", "Playback"})  [unwired: 1 in]
        n246 = global write "WPI_DashboardLogging Global.vi" "Logging Filename"(path "") -> ()
        n247 = case shown="\"Stop\", \"Record\"" w392 {
          tunnel: w391 -> [_ w394 w402]
          tunnel: [_ _ w401] -> w388
          tunnel: [_ _ w400] -> _
          tunnel: w386 -> [_ _ w398]
          tunnel: cluster{i32, i32} {-250, 170} -> [_ _ w397]
          tunnel: [_ _ T15 {"Image Size"=TRUE, "Image Type"=TRUE, "Pixel Value"=TRUE, "ROI Information"=TRUE, "Zoom Factor"=FALSE} ("Image Information Shown:All Elements")] -> w384
          tunnel: [_ _ TRUE ("Zoom Factor")] -> w383
          frame Default {
          }
          frame "Stop", "Record" {
            # "Place Window too"
            n248 = invoke class="VI" method="FP.Close"(reference=w394) -> (reference out=w393:refnum<vi>)  [unwired: 2 in, 2 out]
            n249 = invoke class="VI" method="Abort VI"(reference=w393) -> ()  [unwired: 2 in, 3 out]
          }
          frame "Playback" {
            n250 = call "Open Playback Panel.vi"("Offset"=w397, "DB VI Ref"=w398, "Playback in"=w402) -> ("Playback out"=w399:refnum<vi>)  [unwired: 8 in]
            n251 = register-events(w399) -> (reference out=w401:refnum<event-registration>, error out=w400:errorcluster)  [unwired: 2 in]
          }
        }
        n252 = global write "WPI_DashboardLogging Global.vi" "Recording"(w392) -> ()
        n253 = property on="Camera Image" class="ImageControl"("Image Information Shown"=w384, "Image Information Visible"=w383) -> ()  [unwired: 2 in, 2 out]
        n254 = call <vilib>:"WPI_DashboardNT Log FieldName Cache.vi"("Operation"=enum16{"Lookup/Add", "Index", "Clear"}."Clear") -> ()  [unwired: 8 in, 3 out]
      }
      event Panel Close {
        w403 = enum32{"Stop", "Record", "Playback"}."Stop" ("Rec Mode")
        n255 = event-data() -> ()  [unwired: 1 in, 4 out]
        n256 = local write "Rec Mode"(w403) -> ()
        n257 = global write "WPI_DashboardLogging Global.vi" "Recording"(w403) -> ()
      }
      event Panel Close {
        # "Abort playback window and ourself"
        n258 = event-data() -> ()  [unwired: 1 in, 4 out]
        n259 = invoke class="VI" method="FP.Close"(reference=w408) -> (reference out=w407:refnum<vi>)  [unwired: 2 in, 2 out]
        n260 = invoke class="VI" method="Abort VI"(reference=w407) -> (error out=w406:errorcluster)  [unwired: 2 in, 2 out]
        n261 = invoke class="VI" method="Abort VI"(error in=w406) -> ()  [unwired: 2 in, 3 out]
      }
    }
  }
  n262 = property on="On/Off" class="Bool (strict)"("Visible"=w27) -> ()  [unwired: 2 in, 2 out]
  n263 = property on="Motor" class="Clust (strict)"("Visible"=w27) -> ()  [unwired: 2 in, 2 out]
  n264 = property on="Progress" class="Clust (strict)"("Visible"=w27) -> ()  [unwired: 2 in, 2 out]
  n265 = property on="Test Ring" class="Ring (strict)"("Visible"=w27) -> ()  [unwired: 2 in, 2 out]
  n266 = property on="Rev/Fwd" class="Clust (strict)"("Visible"=w27) -> ()  [unwired: 2 in, 2 out]
  n267 = property on="Camera Settings" class="Clust (strict)"("Visible"=w27) -> ()  [unwired: 2 in, 2 out]
  n268 = local write "DB Camera Config"(w27) -> ()
  n269 = global write "WPI_DashboardLogging Global.vi" "Recording"(w10) -> ()
  n270 = local write "Rec Mode"(w10) -> ()
  n271 = call <vilib>:"SD Write Number.vi"("Numeric"="Throttle", "Name"="Throttle") -> ()  [unwired: 8 in, 2 out]
